vi "Initialize Sensors B.vi"(11 "?":T1={"     Use ?\nOff       On"=[FALSE, TRUE, FALSE, TRUE], "Mode:"=FALSE, "Rx Prop Port"="", "Hokuyo Port"="COM7", "Tx Prop  Port"="COM6", "Compass Port"="", "GPS Port"=""}) -> (3 "?":T1={"     Use ?\nOff       On"=[FALSE, TRUE, FALSE, TRUE], "Mode:"=FALSE, "Rx Prop Port"="", "Hokuyo Port"="COM7", "Tx Prop  Port"="COM6", "Compass Port"="", "GPS Port"=""})   [LabVIEW 2014]
uses:
  Initialize-Standard.vi
  Hokuyo URG Series.lvlib
panel:
  in  "Checksum":bool
  in  "ID Query?":bool=TRUE
  in  "Protocol":u32(ring)=2 items=["Convert to Latest", "SCIP 1.1", "SCIP 2.0"]
  # "Initialize Sensors B"
  # "Input:"
  # "Output:"
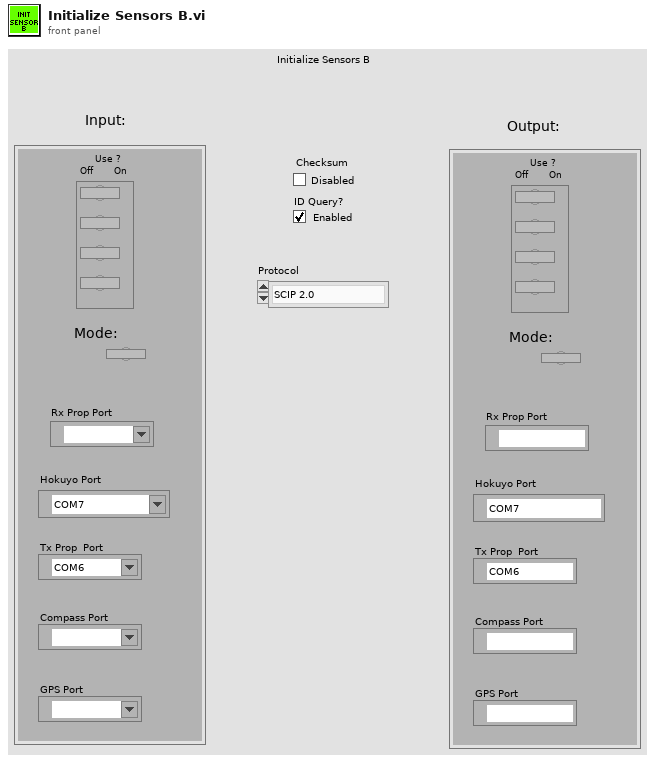
[diagram p1: front panel]
types:
  T1 = cluster{"     Use ?\nOff       On":bool[], "Mode:":bool, "Rx Prop Port":refnum<visa-resource-name>, "Hokuyo Port":refnum<visa-resource-name>, "Tx Prop  Port":refnum<visa-resource-name>, "Compass Port":refnum<visa-resource-name>, "GPS Port":refnum<visa-resource-name>}
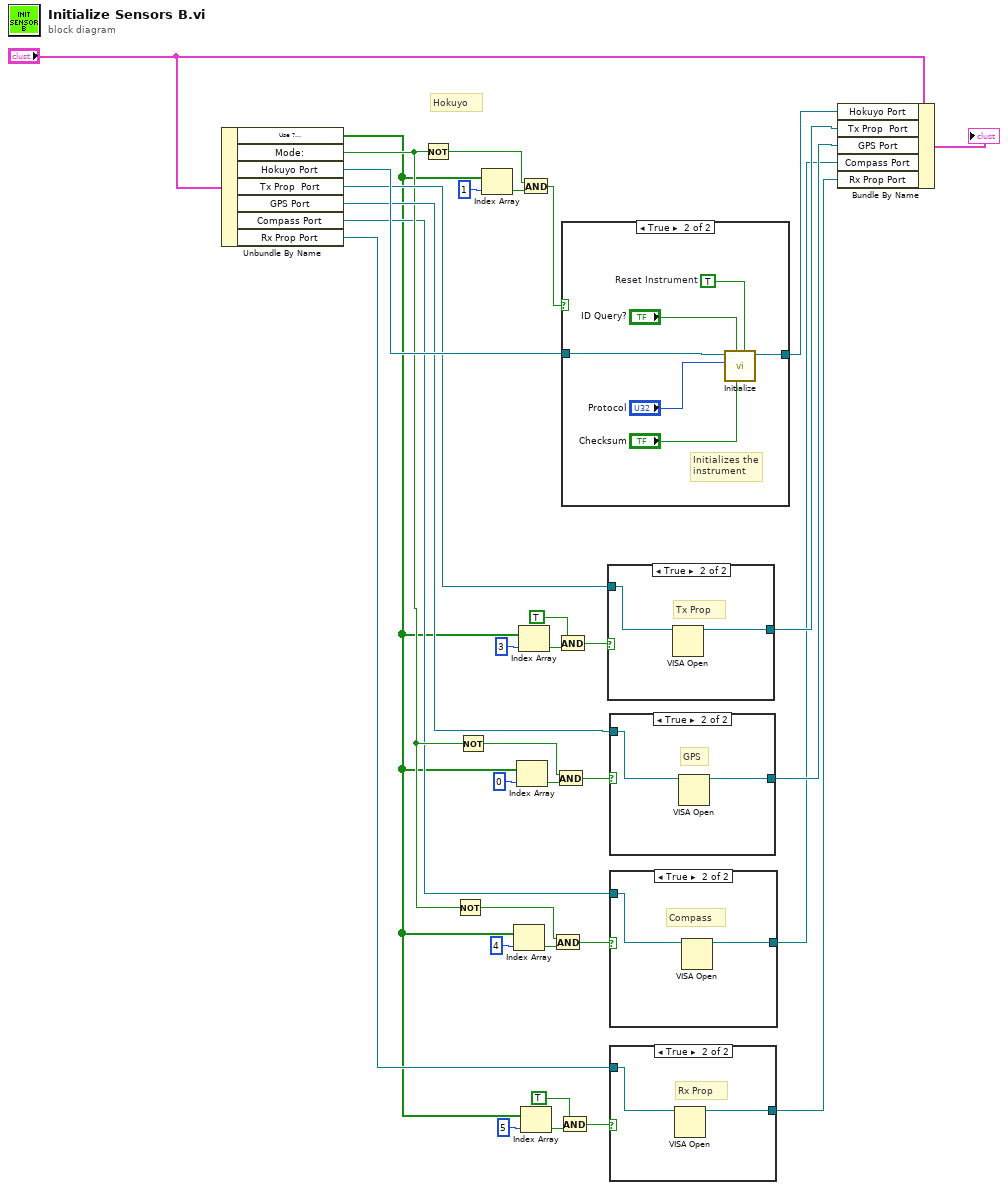
[diagram p0: block diagram]
diagram:
  # "Hokuyo"
  n1 = Unbundle By Name("?") -> ("Use ?\nOff       On"=w2:bool[], "Mode:"=w11:bool, "Hokuyo Port"=w31:refnum<visa-resource-name>, "Tx Prop  Port"=w23:refnum<visa-resource-name>, "GPS Port"=w17:refnum<visa-resource-name>, "Compass Port"=w10:refnum<visa-resource-name>, "Rx Prop Port"=w3:refnum<visa-resource-name>)
  n2 = Not(x=w11) -> (.not. x?=w32:bool)
  n3 = Not(x=w11) -> (.not. x?=w13:bool)
  n4 = Not(x=w11) -> (.not. x?=w19:bool)
  n5 = Index Array(array=w2, index=1) -> (element=w33:bool)
  n6 = Index Array(array=w2, index=4) -> (element=w14:bool)
  n7 = Index Array(array=w2, index=0) -> (element=w20:bool)
  n8 = Index Array(array=w2, index=3) -> (element=w25:bool)
  n9 = And(x=w32, y=w33) -> (x .and. y?=w30:bool)
  n10 = Index Array(array=w2, index=5) -> (element=w6:bool)
  n11 = And(x=w13, y=w14) -> (x .and. y?=w12:bool)
  n12 = And(x=w19, y=w20) -> (x .and. y?=w18:bool)
  n13 = And(x=TRUE, y=w25) -> (x .and. y?=w24:bool)
  n14 = And(x=TRUE, y=w6) -> (x .and. y?=w5:bool)
  n15 = case shown="True" w30 {
    tunnel: w31 -> [w35 w37]
    tunnel: [w35 w36] -> w29
    frame False {
    }
    frame True {
      w39 = TRUE  # Reset Instrument
      # "Initializes the instrument"
      n16 = call-poly "Initialize.vi"("Reset? (F: No)"=w39, "Checksum (Disabled)"="Checksum", "ID Query? (Enabled)"="ID Query?", "Protocol (2: SCIP 2.0)"="Protocol", "VISA resource name"=w37) -> ("VISA resource name out"=w36:refnum<visa-resource-name>)  [unwired: 5 in, 1 out]
    }
  }
  n17 = case shown="True" w24 {
    tunnel: w23 -> [w42 w44]
    tunnel: [w42 w43] -> w22
    frame False {
    }
    frame True {
      # "Tx Prop"
      n18 = VISA Open(VISA resource name=w44) -> (VISA resource name=w43:refnum<visa-resource-name>)  [unwired: 4 in, 1 out]
    }
  }
  n19 = case shown="True" w18 {
    tunnel: w17 -> [w45 w47]
    tunnel: [w45 w46] -> w16
    frame False {
    }
    frame True {
      # "GPS"
      n20 = VISA Open(VISA resource name=w47) -> (VISA resource name=w46:refnum<visa-resource-name>)  [unwired: 4 in, 1 out]
    }
  }
  n21 = case shown="True" w12 {
    tunnel: w10 -> [w48 w50]
    tunnel: [w48 w49] -> w9
    frame False {
    }
    frame True {
      # "Compass"
      n22 = VISA Open(VISA resource name=w50) -> (VISA resource name=w49:refnum<visa-resource-name>)  [unwired: 4 in, 1 out]
    }
  }
  n23 = case shown="True" w5 {
    tunnel: w3 -> [w51 w53]
    tunnel: [w51 w52] -> w1
    frame False {
    }
    frame True {
      # "Rx Prop"
      n24 = VISA Open(VISA resource name=w53) -> (VISA resource name=w52:refnum<visa-resource-name>)  [unwired: 4 in, 1 out]
    }
  }
  n25 = Bundle By Name(cluster="?", "Hokuyo Port"=w29, "Tx Prop  Port"=w22, "GPS Port"=w16, "Compass Port"=w9, "Rx Prop Port"=w1) -> (→"?":T1)
